vi "Find_Data_SubVI.vi"(0 "FGGA":string, 5 "CO":string, 7 "Ozone":string, 9 "SO2":string) -> (4 "Output Value":dbl)   [LabVIEW 2014]
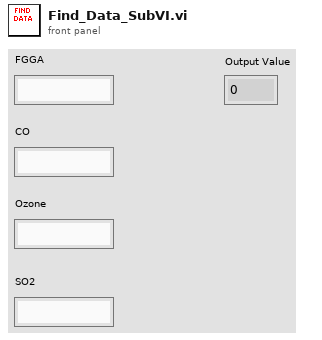
[diagram p1: front panel]
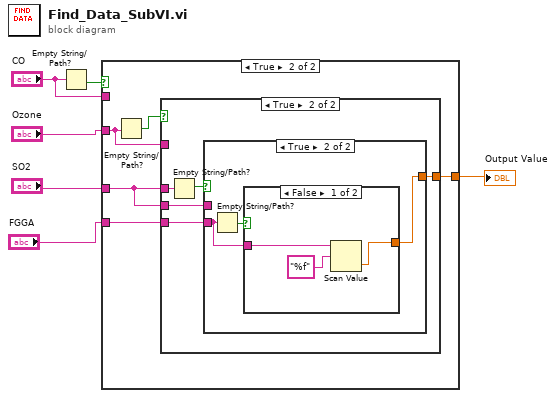
[diagram p0: block diagram]
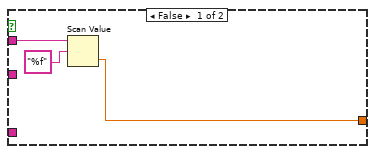
[diagram p2: hidden frame]
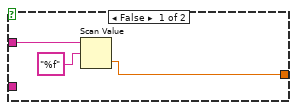
[diagram p3: hidden frame]
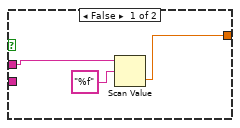
[diagram p4: hidden frame]
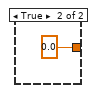
[diagram p5: hidden frame]
diagram:
  n1 = Empty String/Path?(string/path="CO") -> (empty?=w6:bool)
  n2 = case shown="True" w6 {
    tunnel: "CO" -> [w8 _]
    tunnel: [w7 w13] -> w5
    tunnel: "Ozone" -> [_ w10]
    tunnel: "SO2" -> [_ w11]
    tunnel: "FGGA" -> [_ w12]
    frame False {
      n3 = Scan Value(string=w8, format string="%f") -> (value=w7:dbl)  [unwired: 1 in, 1 out]
    }
    frame True {
      n4 = Empty String/Path?(string/path=w10) -> (empty?=w14:bool)
      n5 = case shown="True" w14 {
        tunnel: w10 -> [w16 _]
        tunnel: w11 -> [_ w22]
        tunnel: [w15 w18] -> w13
        tunnel: w12 -> [_ w20]
        tunnel: w11 -> [_ w19]
        frame False {
          n6 = Scan Value(string=w16, format string="%f") -> (value=w15:dbl)  [unwired: 1 in, 1 out]
        }
        frame True {
          n7 = Empty String/Path?(string/path=w22) -> (empty?=w21:bool)
          n8 = case shown="True" w21 {
            tunnel: w20 -> [_ w26]
            tunnel: w19 -> [w24 _]
            tunnel: [w23 w27] -> w18
            frame False {
              n9 = Scan Value(string=w24, format string="%f") -> (value=w23:dbl)  [unwired: 1 in, 1 out]
            }
            frame True {
              n10 = Empty String/Path?(string/path=w26) -> (empty?=w28:bool)
              n11 = case shown="False" w28 {
                tunnel: [w29 0.0] -> w27
                tunnel: w26 -> [w30 _]
                frame False {
                  n12 = Scan Value(string=w30, format string="%f") -> (value=w29:dbl)  [unwired: 1 in, 1 out]
                }
                frame True {
                }
              }
            }
          }
        }
      }
    }
  }
  "Output Value" <- w5
